vi "(SubVI) XY information for Stage and DAQ channel_YCC.vi"(5 "T=X\nF=Y":bool) -> (1 "physical channels":tag, 2 "Axis":i32)   [LabVIEW 2014]
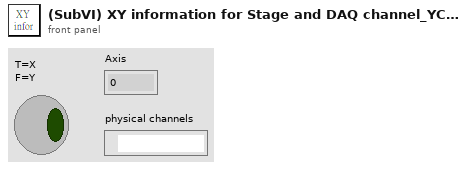
[diagram p1: front panel]
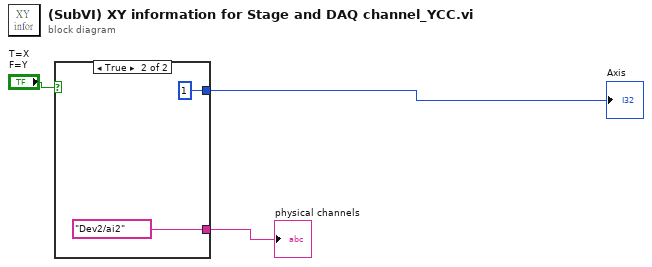
[diagram p0: block diagram]
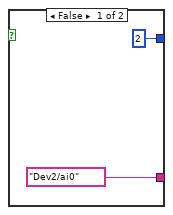
[diagram p2: hidden frame]
diagram:
  n1 = case shown="True" "T=X\nF=Y" {
    tunnel: [2 1] -> w2
    tunnel: [tag "Dev2/ai0" ("physical channels") tag "Dev2/ai2" ("physical channels")] -> w3
    frame False {
    }
    frame True {
    }
  }
  "physical channels" <- w3
  "Axis" <- w2
